vi "CAN_Recive.vi"(8 "error in (no error)":errorcluster, 9 "T?R":bool, 10 "CAN_OBJ_RN":T1[](array[typedef]), 11 "NUM":u16) -> (0 "error out":errorcluster)   [LabVIEW 2020, in "ZLG_CAN.lvlib"]
doc: "_____\nCreated using Delacor QMH Event Scripter 4.1.0.80."
uses:
  ZLG_CAN.lvlib
  CAN_OBJ_R.ctl
  CAN_Recive Argument--cluster.ctl
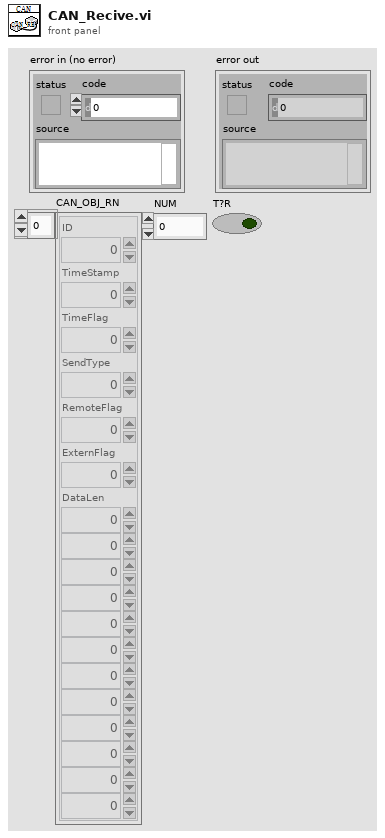
[diagram p1: front panel]
types:
  T1 = typedef "ZLG_CAN.lvlib/CAN_OBJ_R.ctl" = cluster{"ID":u32, "TimeStamp":u32, "TimeFlag":u8, "SendType":u8, "RemoteFlag":u8, "ExternFlag":u8, "DataLen":u8, "数值":u8, "数值":u8, "数值":u8, "数值":u8, "数值":u8, "数值":u8, "数值":u8, "数值":u8, "数值":u8, "数值":u8, "数值":u8}
  T2 = typedef "ZLG_CAN.lvlib/CAN_Recive Argument--cluster.ctl" = cluster{"T?R":bool, "NUM":u16, "CAN_OBJ_RN":T1[]}
  T3 = typedef "ZLG_CAN.lvlib/Broadcast Events--cluster.ctl" = cluster{"Module Did Init":refnum<user-event>, "Status Updated":refnum<user-event>, "Error Reported":refnum<user-event>, "Module Did Stop":refnum<user-event>, "Update Module Execution Status":refnum<user-event>, "CAN_Recive":refnum<user-event>}
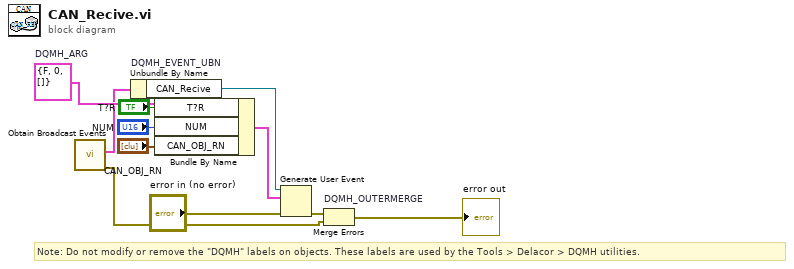
[diagram p0: block diagram]
diagram:
  w6 = T2 {"T?R"=FALSE, "NUM"=0, "CAN_OBJ_RN"=[]}  # DQMH_ARG
  # "Note: Do not modify or remove the \"DQMH\" labels on objects. These labels are used by the Tools > Delacor > DQMH utilities."
  n1 = call "Obtain Broadcast Events.vi"() -> ("error out"=w5:errorcluster, "ZLG_CAN Broadcast Events"=w4:T3)  [unwired: 10 in]
  n2 = Unbundle By Name "DQMH_EVENT_UBN"(w4) -> ("CAN_Recive"=w8:refnum<user-event>)
  n3 = Bundle By Name ("DQMH_BBN")(cluster=w6, "T?R"="T?R", "NUM"="NUM", "CAN_OBJ_RN"="CAN_OBJ_RN") -> (w9:T2)
  n4 = Generate User Event(user event=w8, event data cluster=w9, error in="error in (no error)") -> (error out=w7:errorcluster)  [unwired: 1 in, 1 out]
  n5 = Merge Errors "DQMH_OUTERMERGE"(w7, w5) -> (→"error out":errorcluster)
